vi "时间日期字符串转换为时间格式.vi"(8 "error in (no error)":errorcluster caption="错误输入（无错误）", 11 "时间日期字符串":string="2018/10/23 11:48:48") -> (0 "error out":errorcluster caption="错误输出", 3 "时间标识":timestamp)   [LabVIEW 2016]
uses:
  <vilib>/Utility/miscctls.llb/LVDateTimeRec.ctl
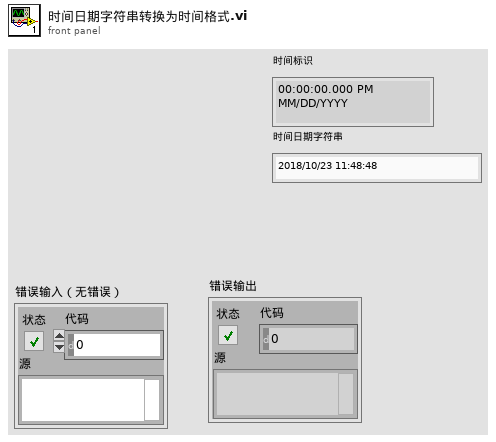
[diagram p1: front panel]
types:
  T1 = typedef "LVDateTimeRec.ctl" = cluster{"fractional second":dbl, "second":i32, "minute":i32, "hour":i32, "day of month":i32, "month":i32, "year":i32, "day of week":i32, "day of year":i32, "DST":i32}
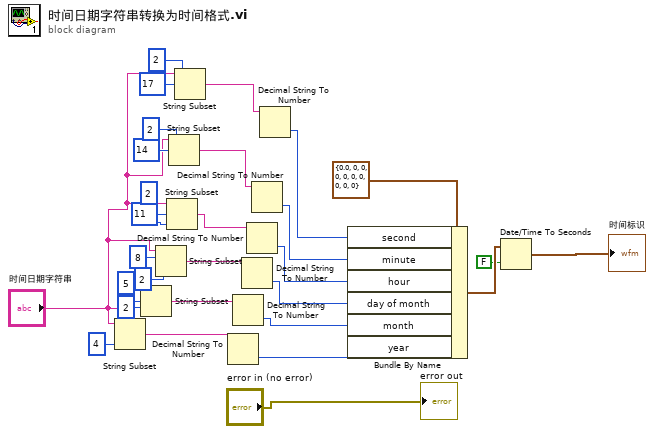
[diagram p0: block diagram]
diagram:
  n1 = String Subset(string="时间日期字符串", length (rest)=4 ("长度（剩余）")) -> (substring=w25:string)  [unwired: 1 in]
  n2 = String Subset(string="时间日期字符串", offset (0)=5 ("偏移量(0)"), length (rest)=2 ("长度（剩余）")) -> (substring=w22:string)
  n3 = String Subset(string="时间日期字符串", offset (0)=8 ("偏移量(0)"), length (rest)=2 ("长度（剩余）")) -> (substring=w17:string)
  n4 = String Subset(string="时间日期字符串", offset (0)=11 ("偏移量(0)"), length (rest)=2 ("长度（剩余）")) -> (substring=w14:string)
  n5 = String Subset(string="时间日期字符串", offset (0)=14 ("偏移量(0)"), length (rest)=2 ("长度（剩余）")) -> (substring=w9:string)
  n6 = String Subset(string="时间日期字符串", offset (0)=17 ("偏移量(0)"), length (rest)=2 ("长度（剩余）")) -> (substring=w4:string)
  n7 = Decimal String To Number(string=w25) -> (number=w24:i32)  [unwired: 2 in, 1 out]
  n8 = Decimal String To Number(string=w22) -> (number=w21:i32)  [unwired: 2 in, 1 out]
  n9 = Decimal String To Number(string=w17) -> (number=w16:i32)  [unwired: 2 in, 1 out]
  n10 = Decimal String To Number(string=w14) -> (number=w13:i32)  [unwired: 2 in, 1 out]
  n11 = Decimal String To Number(string=w9) -> (number=w8:i32)  [unwired: 2 in, 1 out]
  n12 = Decimal String To Number(string=w4) -> (number=w3:i32)  [unwired: 2 in, 1 out]
  n13 = Bundle By Name(cluster=T1 {"fractional second"=0.0, "second"=0, "minute"=0, "hour"=0, "day of month"=0, "month"=0, "year"=0, "day of week"=0, "day of year"=0, "DST"=0} ("日期时间记录"), "second"=w3, "minute"=w8, "hour"=w13, "day of month"=w16, "month"=w21, "year"=w24) -> (w28:T1)
  n14 = Date/Time To Seconds(1:FALSE ("是UTC (F)"), 2:w28) -> (0:→"时间标识":timestamp)
  "error out" <- "error in (no error)"
